vi "Set Slave ID.vi"(8 "error in (no error)":errorcluster, 10 "Slave ID":u8=1, 11 "MB PLC in":refnum<class "MB PLC Client.lvclass">) -> (0 "error out":errorcluster, 3 "MB PLC out":refnum<class "MB PLC Client.lvclass">)   [LabVIEW 2018, in "MB PLC Client.lvlib" / "MB PLC Client.lvclass"]
uses:
  MB PLC Client.lvclass
  MB PLC Client.lvclass/MB PLC Client.ctl
  <vilib>/Plasmionique/MB Master/MB_Master/MB_Master.lvclass
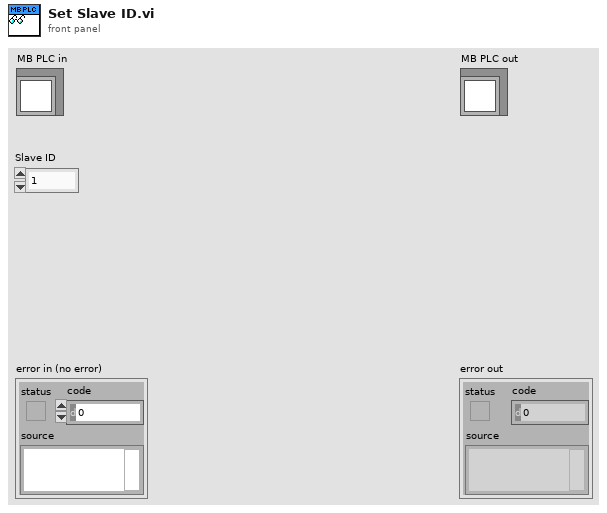
[diagram p1: front panel]
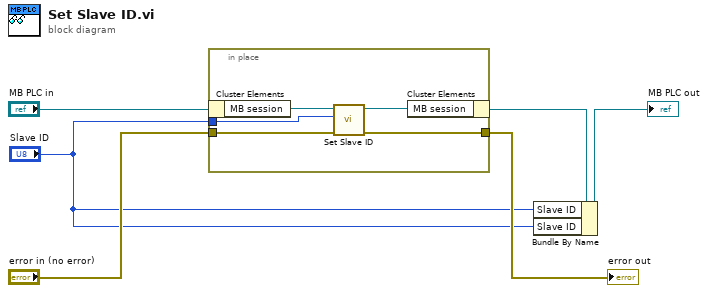
[diagram p0: block diagram]
diagram:
  n1 = in-place {
    in-place-border: "error in (no error)" -> [w9]
    in-place-border: [w8] -> w4
    in-place-border: "Slave ID" -> [w7]
    n2 = in-place-cluster #1("MB PLC in") -> ("MB session"=w11:refnum<class "MB_Master.lvclass">)
    n3 = call-dynamic "Set Slave ID.vi"("error in (no error)"=w9, "Slave ID"=w7, "MB_Master in"=w11) -> ("error out"=w8:errorcluster, "MB_Master out"=w10:refnum<class "MB_Master.lvclass">)  [unwired: 7 in]
    n4 = in-place-cluster #1("MB session"=w10) -> (w3:refnum<class "MB PLC Client.lvclass">)
  }
  "error out" <- w4
  n5 = Bundle By Name(cluster=w3, "Slave ID"="Slave ID", "Slave ID"="Slave ID") -> (→"MB PLC out":refnum<class "MB PLC Client.lvclass">)
